vi "LimitAcceleration.vi"(1 "Apply Limit":bool, 2 "Decceleration Limit (/s)":dbl, 3 "Acceleration Limit (/s)":dbl, 4 "Raw Input":dbl) -> (0 "Output":dbl)   [LabVIEW 2019]
doc: "This VI modifies the raw input with acceleration/decceleration limits. Please use the built-in toggle capability if switching between limited and unlimited modes, otherwise unexpected output behavior could occur."
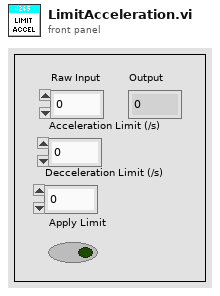
[diagram p1: front panel]
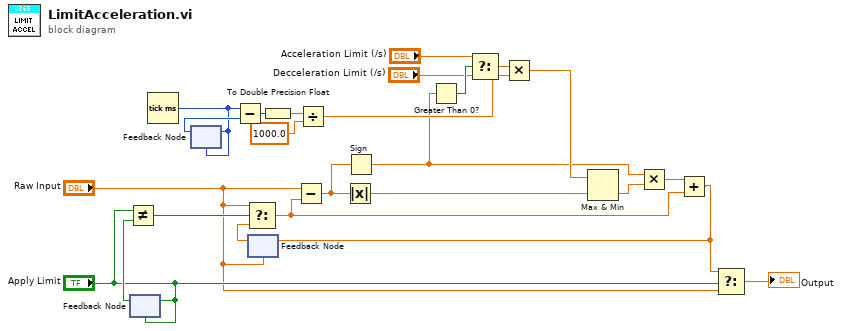
[diagram p0: block diagram]
diagram:
  n1 = feedback-in #1("Apply Limit") -> ()
  n2 = feedback #1("Apply Limit") -> (w6:bool)
  n3 = Not Equal?(x="Apply Limit", y=w6) -> (x != y?=w4:bool)
  n4 = Tick Count (ms)() -> (millisecond timer value=w19:u32)
  n5 = feedback-in #2(w19) -> ()
  n6 = feedback #2(w19) -> (w20:u32)
  n7 = Subtract(x=w19, y=w20) -> (x-y=w18:u32)
  n8 = feedback #3("Raw Input") -> (w3:dbl)
  n9 = Select(t="Raw Input", s=w4, f=w3) -> (s? t:f=w2:dbl)
  n10 = To Double Precision Float(number=w18) -> (double precision float=w16:dbl)
  n11 = Subtract(x="Raw Input", y=w2) -> (x-y=w24:dbl)
  n12 = Divide(x=w16, y=1000.0) -> (x/y=w15:dbl)
  n13 = Absolute Value(x=w24) -> (abs(x)=w23:dbl)
  n14 = Sign(1:w24) -> (0:w12:dbl)
  n15 = Greater Than 0?(x=w12) -> (x > 0?=w11:bool)
  n16 = Select(t="Acceleration Limit (/s)", s=w11, f="Decceleration Limit (/s)") -> (s? t:f=w13:dbl)
  n17 = Multiply(x=w13, y=w15) -> (x*y=w17:dbl)
  n18 = Max & Min(x=w17, y=w23) -> (min(x,y)=w22:dbl)  [unwired: 1 out]
  n19 = Multiply(x=w12, y=w22) -> (x*y=w21:dbl)
  n20 = Add(x=w21, y=w2) -> (x+y=w8:dbl)
  n21 = feedback-in #3(w8) -> ()
  n22 = Select(t=w8, s="Apply Limit", f="Raw Input") -> (s? t:f=→"Output":dbl)
